vi "yolo-version.vi"() -> ()   [LabVIEW 2017]
uses:
  <vilib>/LVH/i3 JSON/JSON Parsing/Get Object Parameter Files/Get Object Parameter - String.vi
  <vilib>/httpClient/LabVIEWHTTPClient.lvlib
  <vilib>/LVH/i3 JSON/i3-json.lvlib
panel:
  out "version":string
  out "body":string
  out "headers":string
  in  "error in (no error)":errorcluster
  in  "yolo-server \"version \"endpoint":string="http://localhost:18080/version"
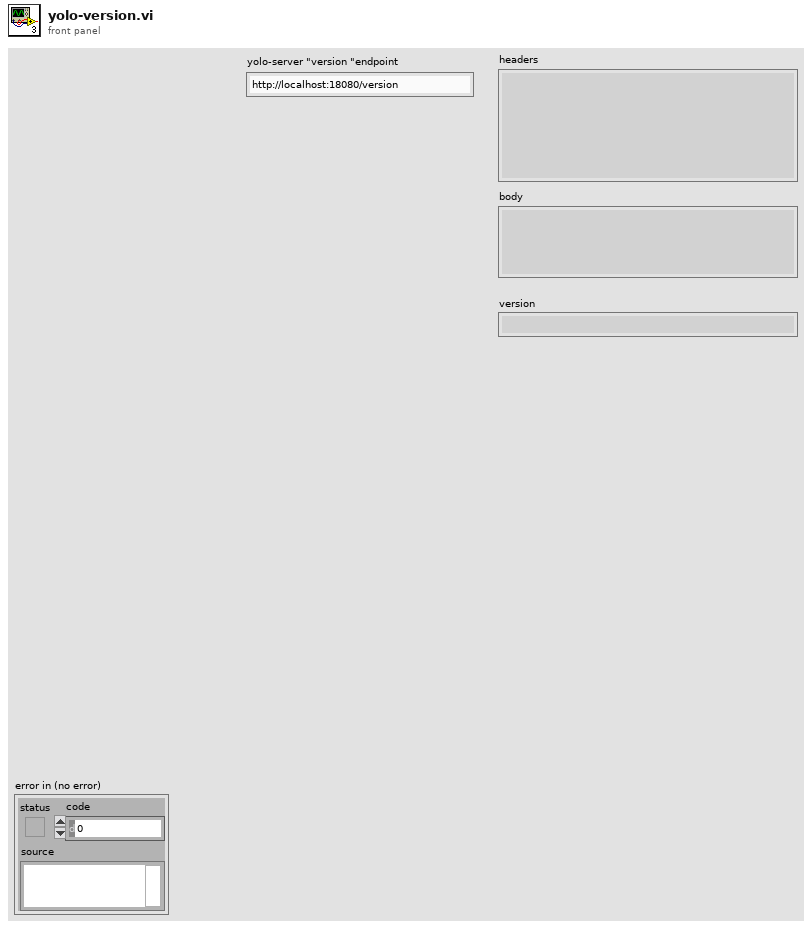
[diagram p1: front panel]
types:
  T1 = typedef "LabVIEWHTTPClient.lvlib/ClientHandle.ctl" = refnum<k1>
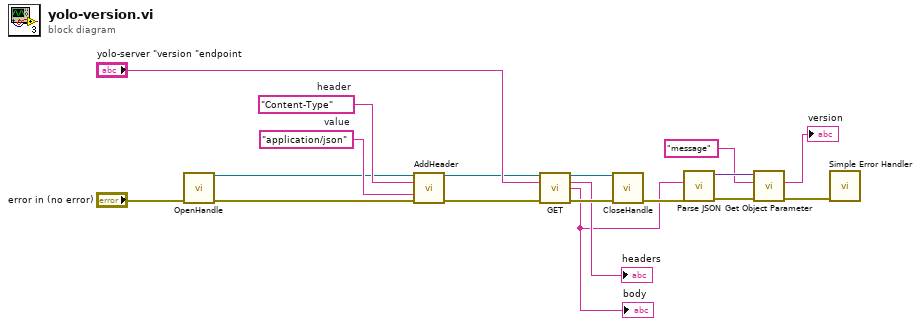
[diagram p0: block diagram]
diagram:
  w18 = "application/json"  # value
  w17 = "Content-Type"  # header
  n1 = call <vilib>:"OpenHandle.vi"("error in (no error)"="error in (no error)") -> ("client handle out"=w9:T1, "error out"=w10:errorcluster)  [unwired: 13 in]
  n2 = call <vilib>:"AddHeader.vi"("client handle"=w9, "header"=w17, "value"=w18, "error in (no error)"=w10) -> ("client handle out"=w11:T1, "error out"=w12:errorcluster)  [unwired: 10 in]
  n3 = call <vilib>:"GET.vi"("client handle"=w11, "url"="yolo-server \"version \"endpoint", "error in (no error)"=w12) -> ("client handle out"=w13:T1, "headers"=→"headers":string, "body"=w6:string, "error out"=w14:errorcluster)  [unwired: 9 in]
  "body" <- w6
  n4 = call <vilib>:"CloseHandle.vi"("client handle"=w13, "error in (no error)"=w14) -> ("error out"=w7:errorcluster)  [unwired: 13 in]
  n5 = call <vilib>:"Parse JSON.vi"("error in (no error)"=w7, "JSON String"=w6) -> ("error out"=w4:errorcluster, "JSON Tree"=w5:variant)  [unwired: 6 in, 2 out]
  n6 = call-poly <vilib>:"Get Object Parameter.vi"("error in (no error)"=w4, "Parameter Name"="message", "JSON Tree In (JSON Object)"=w5) -> ("error out"=w1:errorcluster, "String Value"=→"version":string)  [unwired: 5 in, 2 out]
  n7 = call <vilib>:"Simple Error Handler.vi"("error in (no error)"=w1) -> ()  [unwired: 4 in, 5 out]
